vi "ValidDragDrop.vi"(8 "error in":errorcluster, 10 "drag over":string, 11 "tree ref in":refnum<vi>) -> (0 "error out":errorcluster, 1 "accepted":bool, 2 "drag":string, 3 "tree ref out":refnum<vi>)   [LabVIEW 2013, in "NISE_CEF_TreeControl.lvlib"]
doc: "This VI is used to see if a drag and drop operation is valid.\nThe drop shoudl be done in a node that accepts that kind of nodes."
uses:
  NISE_CEF_TreeControl.lvlib
  Node/NISE_CEF_Node.lvclass
  Node/SubNodeCluster.ctl
  Node/ReadNodeClass.vi
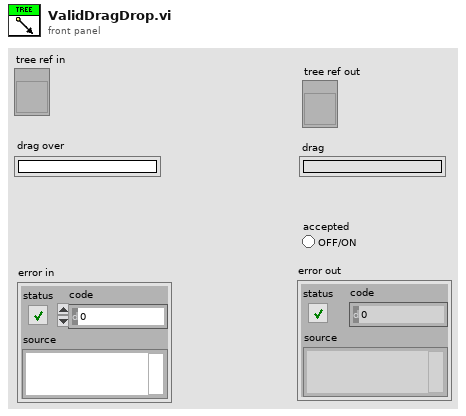
[diagram p1: front panel]
types:
  T1 = typedef "NISE_CEF_Node.lvclass/NodeRef.ctl" = refnum<data-value>
  T2 = typedef "NISE_CEF_Node.lvclass/SubNodeCluster.ctl" = cluster{"subnodes menu name":string[], "subnodes class":string[]}
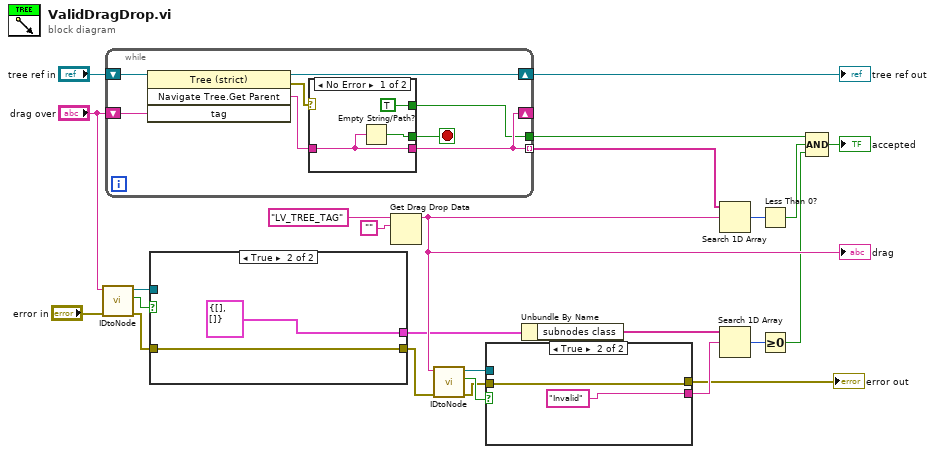
[diagram p0: block diagram]
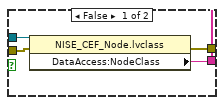
[diagram p2: hidden frame]
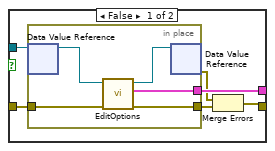
[diagram p3: hidden frame]
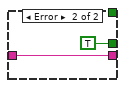
[diagram p4: hidden frame]
diagram:
  n1 = call "IDtoNode.vi"("error in"="error in", "ID"="drag over") -> ("error out"=w5:errorcluster, "invalid Id"=w7:bool, "node ref"=w13:T1)  [unwired: 7 in]
  n2 = while {
    shift-right: [w28] -> _
    shift-left: "drag over" -> [w32]
    tunnel: [w28] -> w22 mode=indexing
    tunnel: [w27] -> w19
    shift-right: [w26] -> w20
    shift-left: "tree ref in" -> [w33]
    stop <- w31 stop-if-true
    n3 = invoke class="Tree (strict)" method="Navigate Tree.Get Parent"(reference=w33, "tag"=w32) -> (reference out=w26:refnum<vi>, error out=w30:errorcluster, "Navigate Tree:Get Parent"=w29:string)  [unwired: 2 in, 1 out]
    n4 = case shown="No Error" w30 {
      tunnel: [w34 TRUE] -> w31
      tunnel: w29 -> [w35 w37]
      tunnel: [w35 w37] -> w28
      tunnel: [TRUE _] -> w27
      frame No Error {
        n5 = Empty String/Path?(string/path=w35) -> (empty?=w34:bool)
      }
      frame Error {
      }
    }
  }
  "tree ref out" <- w20
  n6 = case shown="True" w7 {
    tunnel: w13 -> [w44 _]
    tunnel: [w43 T2 {"subnodes menu name"=[], "subnodes class"=[]} ("subnodes class")] -> w9
    tunnel: w5 -> [w42 w50]
    tunnel: [w39 w50] -> w4
    frame False {
      n7 = in-place {
        in-place-border: [w47] -> w43
        in-place-border: w42 -> [w46]
        in-place-border: [w45] -> w41
        n8 = in-place-dvr #1(w44) -> (w49:refnum<class "NISE_CEF_Node.lvclass">)  [unwired: 1 out]
        n9 = call-dynamic "EditOptions.vi"("error in"=w46, "node in"=w49) -> ("error out"=w45:errorcluster, "subnodes class"=w47:T2, "node out"=w48:refnum<class "NISE_CEF_Node.lvclass">)  [unwired: 6 in, 1 out]
        n10 = in-place-dvr #1(w48) -> (w40:errorcluster)  [unwired: 1 out]
      }
      n11 = Merge Errors(w40, w41) -> (w39:errorcluster)
    }
    frame True {
    }
  }
  n12 = Get Drag Drop Data(8:"", 9:"LV_TREE_TAG" ("data name")) -> (3:w16:string)  [unwired: 1 in, 1 out]
  "drag" <- w16
  n13 = call "IDtoNode.vi"("error in"=w4, "ID"=w16) -> ("error out"=w3:errorcluster, "invalid Id"=w6:bool, "node ref"=w14:T1)  [unwired: 7 in]
  n14 = case shown="True" w6 {
    tunnel: w14 -> [w55 _]
    tunnel: [w54 "Invalid" ("DataAccess:NodeClass")] -> w10
    tunnel: w3 -> [w53 w56]
    tunnel: [w52 w56] -> w1
    frame False {
      n15 = property class="NISE_CEF_Node.lvclass"(reference=w55, error in=w53) -> (error out=w52:errorcluster, "DataAccess:NodeClass"=w54:string)  [unwired: 1 out]
    }
    frame True {
    }
  }
  "error out" <- w1
  n16 = Unbundle By Name(w9) -> ("subnodes class"=w8:string[])
  n17 = Search 1D Array(1D array=w22, element=w16) -> (index of element=w24:i32)  [unwired: 1 in]
  n18 = Search 1D Array(1D array=w8, element=w10) -> (index of element=w12:i32)  [unwired: 1 in]
  n19 = Less Than 0?(x=w24) -> (x < 0?=w18:bool)
  n20 = Greater Or Equal To 0?(x=w12) -> (x >= 0?=w11:bool)
  n21 = Compound Arithmetic op=AND(w19, w18, w11) -> (→"accepted":bool)
